vi "Get Board Image.vi"(8 "error in (no error)":errorcluster, 10 "Board":string, 11 "Platform in":refnum<class "Platform.lvclass">) -> (0 "error out":errorcluster, 2 "Board Image":picture, 3 "Platform out":refnum<class "Platform.lvclass">)   [LabVIEW 2020, in "PicoG-Core.lvlib" / "Platform.lvclass"]
uses:
  Platform.lvclass
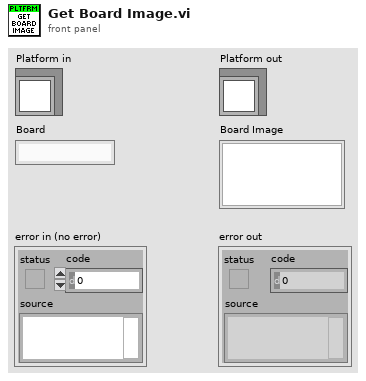
[diagram p1: front panel]
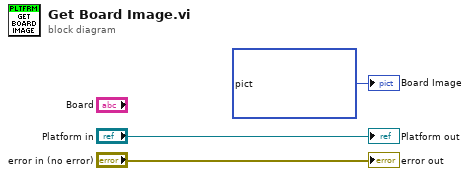
[diagram p0: block diagram]
diagram:
  "error out" <- "error in (no error)"
  "Platform out" <- "Platform in"
  "Board Image" <- picture bytes[22590] ("new picture")
